vi "2015 Winch angle calc.vi"() -> (3 "Winch angle":dbl format="%#_13g")   [LabVIEW 2014]
uses:
  <vilib>/myRIO/Instrument Drivers/Onboard IO/DIO/typedefs/DIO Reference.ctl
  <vilib>/myRIO/Common/Instrument Driver Framework/Utilities/typedefs/myRIO Generic Hardware Reference.ctl
  <vilib>/myRIO/Common/Instrument Driver Framework/Utilities/typedefs/Hardware Version Enum.ctl
  <vilib>/myRIO/Common/Instrument Driver Framework/Utilities/typedefs/myRIO v1.0 Reference.ctl
  <vilib>/myRIO/Common/Instrument Driver Framework/Utilities/typedefs/Generic FPGA Reference.ctl
  <vilib>/myRIO/Common/Instrument Driver Framework/myRIO v1.0/DIO/typedefs/DIO Channels List.ctl
  <vilib>/myRIO/Common/Instrument Driver Framework/myRIO v1.0/DIO/typedefs/DIO Channels Enum.ctl
  <vilib>/userdefined/High Color/nirio_resource_hc.ctl
  <vilib>/myRIO/Instrument Drivers/Onboard IO/DIO/vis/Read.vi
  <vilib>/myRIO/Common/Instrument Driver Framework/myRIO v1.0/DIO/vis/myRIO v1.1 Open DIO.vi
  <vilib>/myRIO/Common/Instrument Driver Framework/Utilities/vis/Is FPGA Ref Available.vi
  <vilib>/myRIO/Common/Instrument Driver Framework/Utilities/vis/Validate Channels.vi
  <vilib>/myRIO/Common/Instrument Driver Framework/myRIO v1.0/DIO/vis/myRIO v1.0 Reserve DIO.vi
  <vilib>/myRIO/Common/Instrument Driver Framework/myRIO v1.0/Resource Manager/vis/myRIO v1.0 Reserve Channel List.vi
  <vilib>/myRIO/Common/Instrument Driver Framework/myRIO v1.0/DIO/vis/myRIO v1.0 Build MUX Configuration DIO.vi
  <vilib>/myRIO/Common/Instrument Driver Framework/myRIO v1.0/Resource Manager/vis/myRIO v1.0 Reserve Channel.vi
  <vilib>/myRIO/Common/Instrument Driver Framework/myRIO v1.0/Resource Manager/vis/myRIO v1.0 Unreserve Channel.vi
  <vilib>/myRIO/Common/Instrument Driver Framework/myRIO v1.0/Resource Manager/vis/myRIO v1.0 Create Configuration List.vi
  <vilib>/myRIO/Common/Instrument Driver Framework/myRIO v1.0/Resource Manager/vis/myRIO v1.0 Build Mutex Name.vi
  <vilib>/myRIO/Common/Instrument Driver Framework/myRIO v1.0/DIO/vis/myRIO v1.0 Read DIO.vi
  <vilib>/Utility/error.llb/Error Cluster From Error Code.vi
  <vilib>/myRIO/Common/Instrument Driver Framework/myRIO v1.0/myRIO v1.0 Close.vi
  <vilib>/myRIO/Common/Instrument Driver Framework/myRIO v1.0/Resource Manager/vis/myRIO v1.0 Configure IO.vi
  <vilib>/myRIO/Common/Instrument Driver Framework/Utilities/vis/IO Manager.vi
  <vilib>/myRIO/Common/Instrument Driver Framework/Utilities/vis/Configuration Manager.vi
  <vilib>/myRIO/Common/Instrument Driver Framework/myRIO v1.0/myRIO v1.1 Open.vi
  <vilib>/Utility/VariantDataType/GetNumericInfo.vi
  <vilib>/myRIO/Instrument Drivers/Onboard IO/DIO/vis/myRIO DIO Open.xnode
  <vilib>/myRIO/Express VI/Onboard IO/DI/DI Express VI.xnode
  <vilib>/myRIO/Instrument Drivers/Onboard IO/DIO/DIO.lvlib
panel:
  out "Numeric 2":dbl format="%#_13g"
  out "Numeric":dbl format="%#_13g"
  out "Past_time_Y":i32
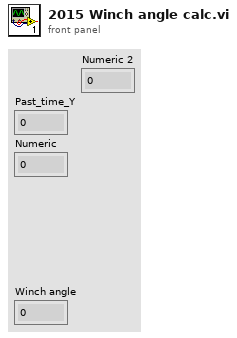
[diagram p1: front panel]
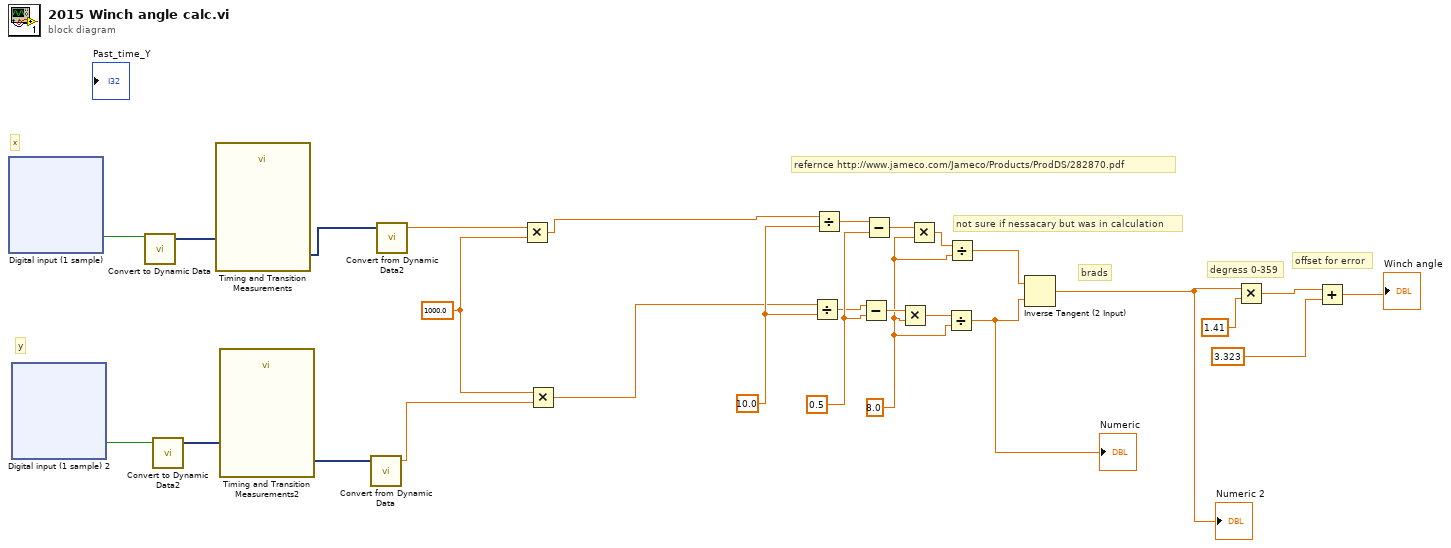
[diagram p0: block diagram]
diagram:
  w5 = 1000.0
  w19 = 8.0
  w26 = 0.5
  w27 = 10.0
  # "offset for error"
  # "y"
  # "x"
  # "degress 0-359"
  # "brads"
  # "refernce http://www.jameco.com/Jameco/Products/ProdDS/282870.pdf"
  # "not sure if nessacary but was in calculation"
  n1 = xnode "Digital input (1 sample)"() -> ("A/DIO8 (Pin 27)"=w11:bool)  [unwired: 1 in, 1 out]
  n2 = xnode "Digital input (1 sample) 2"() -> ("A/DIO9 (Pin 29)"=w8:bool)  [unwired: 1 in, 1 out]
  n3 = call "Convert to Dynamic Data"("Boolean"=w11) -> ("Dynamic Data Type"=w10:dynamicdata)  [unwired: 3 in]
  n4 = call "Convert to Dynamic Data2"("Boolean"=w8) -> ("Dynamic Data Type"=w9:dynamicdata)  [unwired: 3 in]
  n5 = call "Timing and Transition Measurements"("Signals"=w10) -> ("Duration"=w2:dynamicdata)  [unwired: 9 in, 1 out]
  n6 = call "Timing and Transition Measurements2"("Signals"=w9) -> ("Duration"=w1:dynamicdata)  [unwired: 9 in, 1 out]
  n7 = call "Convert from Dynamic Data"("Dynamic Data Type"=w1) -> ("Scalar"=w4:dbl)  [unwired: 3 in]
  n8 = call "Convert from Dynamic Data2"("Dynamic Data Type"=w2) -> ("Scalar"=w3:dbl)  [unwired: 3 in]
  n9 = Multiply(x=w3, y=w5) -> (x*y=w6:dbl)
  n10 = Multiply(x=w5, y=w4) -> (x*y=w7:dbl)
  n11 = Divide(x=w7, y=w27) -> (x/y=w25:dbl)
  n12 = Divide(x=w6, y=w27) -> (x/y=w24:dbl)
  n13 = Subtract(x=w25, y=w26) -> (x-y=w22:dbl)
  n14 = Subtract(x=w24, y=w26) -> (x-y=w23:dbl)
  n15 = Multiply(x=w22, y=w19) -> (x*y=w20:dbl)
  n16 = Multiply(x=w23, y=w19) -> (x*y=w21:dbl)
  n17 = Divide(x=w20, y=w19) -> (x/y=w17:dbl)
  "Numeric" <- w17
  n18 = Divide(x=w21, y=w19) -> (x/y=w18:dbl)
  n19 = Inverse Tangent (2 Input)(1:w17, 2:w18) -> (0:w16:dbl)
  "Numeric 2" <- w16
  n20 = Multiply(x=w16, y=1.41) -> (x*y=w12:dbl)
  n21 = Add(x=w12, y=3.323) -> (x+y=→"Winch angle":dbl)
